vi "Utility_Count Str array.vi"(8 "Error":errorcluster, 11 "String Array":T1) -> (0 "Error Out":errorcluster, 2 "Count Out":i16, 3 "String Array Out":T1)   [LabVIEW 2009]
uses:
  Controls/Array/String Array_Body Text.ctl
  Controls/String_Picture/STRING_Line Display.ctl
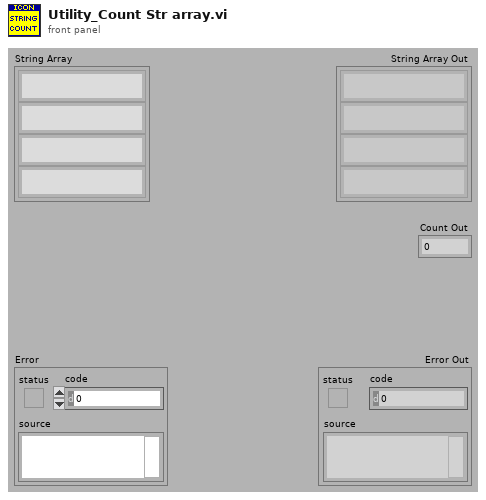
[diagram p1: front panel]
types:
  T1 = typedef "String Array_Body Text.ctl" = T2[]
  T2 = typedef "STRING_Line Display.ctl" = string
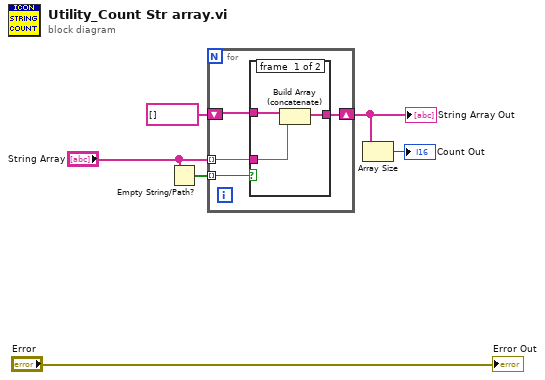
[diagram p0: block diagram]
diagram:
  n1 = Empty String/Path?(string/path="String Array") -> (empty?=w5:bool[])
  n2 = for {
    tunnel: w5 -> [w10] mode=indexing
    tunnel: "String Array" -> [w9] mode=indexing
    shift-right: [w8] -> w2
    shift-left: T2[] [] -> [w7]
    n3 = case shown="True" w10 {
      tunnel: w9 -> [w13 _]
      tunnel: [w12 w14] -> w8
      tunnel: w7 -> [w11 w14]
      frame #0 {
        n4 = Build Array (concatenate)(w11, w13) -> (w12:T2[])
      }
      frame #1 {
      }
    }
  }
  "String Array Out" <- w2
  n5 = Array Size(array=w2) -> (size(s)=→"Count Out":i32)
  "Error Out" <- "Error"
